vi "导出扫描测试数据.vi"(8 "错误输入（无错误）":errorcluster, 10 "数据索引":i32[](array[numeric]), 11 "数组输入":T1[](array[typedef])) -> (0 "错误输出":errorcluster, 2 "数据索引输出":i32[](array[numeric]), 3 "数组输出":T1[](array[typedef]), 5 "扫描数据":dbl[][](array[numeric]), 7 "突变电压":dbl[][](array[numeric]))   [LabVIEW 2021]
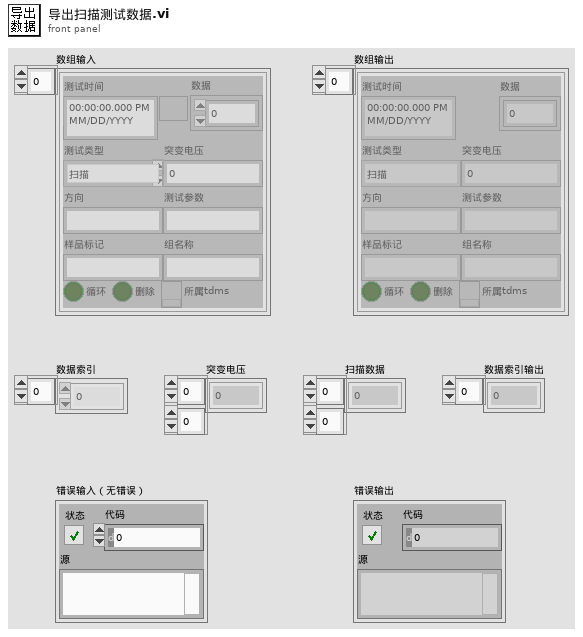
[diagram p1: front panel]
types:
  T1 = typedef "测试数据类型.ctl" = cluster{"测试时间":timestamp, "测试类型":T2, "方向":string, "样品标记":string, "测试参数":string, "循环":bool, "删除":bool, "组名称":string, "所属tdms":refnum<k34>, "突变电压":i32, "数据":dbl[][]}
  T2 = typedef "测试类型.ctl" = enum16{"扫描", "脉冲", "维持时间"}
  T3 = typedef "扫描参数.ctl" = cluster{"测试参数":cluster{"正向电压(V)":dbl, "正向极限电流(mA)":dbl, "反向电压(V)":dbl, "反向极限电流(mA)":dbl}, "时序参数":cluster{"正改变量(V)":dbl, "反改变量(V)":dbl, "维持时间(ms)":dbl, "nplc":dbl, "时序优先":bool}}
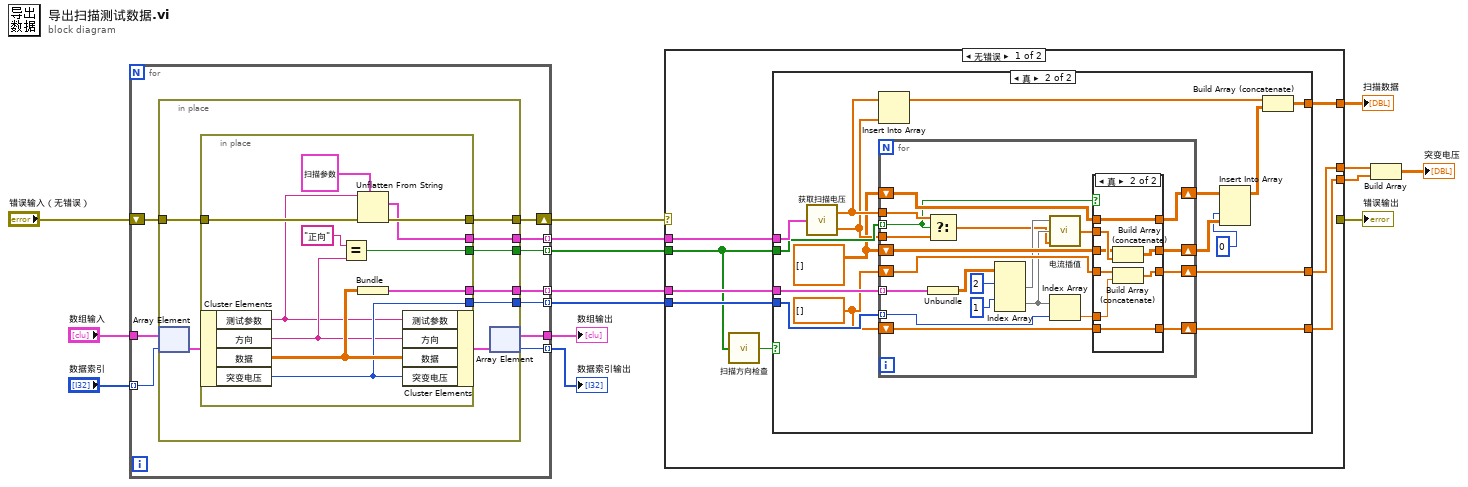
[diagram p0: block diagram]
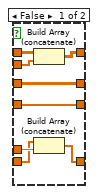
[diagram p3: hidden frame]
diagram:
  n1 = for {
    tunnel: "数据索引" -> [w24] mode=indexing
    tunnel: "数组输入" -> [w25]
    tunnel: [w23] -> w10 mode=indexing
    shift-right: [w21] -> w13
    shift-left: "错误输入（无错误）" -> [w22]
    tunnel: [w20] -> w7 mode=indexing
    tunnel: [w19] -> w8 mode=indexing
    tunnel: [w18] -> w9 mode=indexing
    tunnel: [w17] -> w12
    tunnel: [w16] -> w1 mode=indexing
    n2 = in-place {
      in-place-border: [w31] -> w23
      in-place-border: w22 -> [w30]
      in-place-border: [w29] -> w21
      in-place-border: [w28] -> w20
      in-place-border: [w27] -> w19
      in-place-border: [w26] -> w18
      n3 = in-place-array #1(w25, w24) -> (w33:T1)
      n4 = in-place {
        in-place-border: [w44] -> w31
        in-place-border: w30 -> [w42]
        in-place-border: [w41] -> w29
        in-place-border: [w40] -> w28
        in-place-border: [w37] -> w27
        in-place-border: [w38] -> w26
        n5 = in-place-cluster #2(w33) -> ("测试参数"=w34:string, "方向"=w35:string, "数据"=w39:dbl[][], "突变电压"=w38:i32)
        n6 = Equal?(x="正向" ("y"), y=w35) -> (x = y?=w44:bool)
        n7 = Unflatten From String(type=T3 {"测试参数"={"正向电压(V)"=0.0, "正向极限电流(mA)"=0.0, "反向电压(V)"=0.0, "反向极限电流(mA)"=0.0}, "时序参数"={"正改变量(V)"=0.0, "反改变量(V)"=0.0, "维持时间(ms)"=0.0, "nplc"=0.001, "时序优先"=FALSE}} ("扫描"), binary string=w34, error in (no error)=w42) -> (value=w40:T3, error out=w41:errorcluster)  [unwired: 2 in, 1 out]
        n8 = Bundle("数据"=w39) -> (w37:cluster{"数据":dbl[][]})  [unwired: 1 in]
        n9 = in-place-cluster #2("测试参数"=w34, "方向"=w35, "数据"=w39, "突变电压"=w38) -> (w32:T1)
      }
      n10 = in-place-array #1(w32) -> (w17:T1[], w16:i32)
    }
  }
  "数组输出" <- w12
  "数据索引输出" <- w1
  n11 = case shown="无错误" w13 {
    selector: w13 -> [_ w106]
    tunnel: w7 -> [w52 _]
    tunnel: w8 -> [w51 _]
    tunnel: w9 -> [w50 _]
    tunnel: w10 -> [w49 _]
    tunnel: [w47 _] -> w15
    tunnel: [w46 _] -> w4
    tunnel: [w45 _] -> w3
    tunnel: [_ w106] -> w14
    frame No Error {
      n12 = call "扫描方向检查.vi"("扫描方向"=w49) -> ("检查通过？"=w48:bool)
      n13 = case shown="真" w48 {
        tunnel: w52 -> [_ w68]
        tunnel: w51 -> [_ w67]
        tunnel: w50 -> [_ w66]
        tunnel: w49 -> [_ w65]
        tunnel: [_ w57] -> w47
        tunnel: [_ w56] -> w45
        tunnel: [_ w55] -> w46
        frame False {
        }
        frame True {
          w53 = dbl[] []
          w54 = dbl[][] []
          n14 = call "获取扫描电压.vi"("数组"=w68) -> ("正向扫描电压"=w64:dbl[], "反向扫描电压"=w63:dbl[])
          n15 = Insert Into Array(array=w64, new element=w63) -> (w59:dbl[])  [unwired: 1 in]
          n16 = for {
            tunnel: w67 -> [w89] mode=indexing
            tunnel: w65 -> [w74] mode=indexing
            tunnel: w66 -> [w84] mode=indexing
            tunnel: w64 -> [w86]
            tunnel: w63 -> [w85]
            shift-right: [w83] -> w62
            shift-left: w54 -> [w82]
            shift-right: [w81] -> w60
            shift-left: w54 -> [w80]
            shift-right: [w78] -> w55
            shift-left: w53 -> [w77]
            shift-right: [w76] -> w56
            shift-left: w53 -> [w75]
            n17 = Select(t=w86, s=w74, f=w85) -> (s? t:f=w70:dbl[])
            n18 = Unbundle(w89) -> ("数据"=w73:dbl[][])
            n19 = Index Array(array=w73, index (row) #1=2 ("索引 (行)"), index (row) #2=1 ("索引 (行)")) -> (element #1=w72:dbl[], element #2=w71:dbl[])  [unwired: 2 in]
            n20 = call "电流插值.vi"("电压"=w70, "原始电压"=w71, "原始电流"=w72) -> ("插值后电流"=w69:dbl[])
            n21 = Index Array(array=w71, index=w84) -> (element=w79:dbl)
            n22 = case shown="真" w74 {
              tunnel: w69 -> [w96 w105]
              tunnel: [w97 w104] -> w83
              tunnel: w82 -> [w97 w103]
              tunnel: [w95 w102] -> w81
              tunnel: w80 -> [w94 w102]
              tunnel: w79 -> [w92 w101]
              tunnel: [w93 w100] -> w78
              tunnel: w77 -> [w93 w99]
              tunnel: [w91 w98] -> w76
              tunnel: w75 -> [w90 w98]
              frame False {
                n23 = Build Array (concatenate)(w94, w96) -> (w95:dbl[][])
                n24 = Build Array (concatenate)(w90, w92) -> (w91:dbl[])
              }
              frame True {
                n25 = Build Array (concatenate)(w103, w105) -> (w104:dbl[][])
                n26 = Build Array (concatenate)(w99, w101) -> (w100:dbl[])
              }
            }
          }
          n27 = Insert Into Array(array=w60, index (col)=0 ("索引 (列)"), new element=w62) -> (w58:dbl[][])  [unwired: 1 in]
          n28 = Build Array (concatenate)(w59, w58) -> (w57:dbl[][])
        }
      }
    }
    frame Error {
    }
  }
  "错误输出" <- w14
  "扫描数据" <- w15
  n29 = Build Array(w4, w3) -> (→"突变电压":dbl[][])
